vi "Manual Mode(orig).vi"(5 "slider shoot":dbl, 6 "4 and 5":cluster{"Button 4":bool, "Button 5":bool}, 7 "Shooter":T1, 8 "engage shoot":bool, 9 "Potent":dbl, 11 "Button 1":bool) -> ()   [LabVIEW 2012]
uses:
  <vilib>/Platform/TimedLoop/XDataNode/timing_clust.ctl
  <vilib>/Platform/TimedLoop/XDataNode/nitl_modes.ctl
  <vilib>/Platform/TimedLoop/XDataNode/wakeup.ctl
  <vilib>/Rock Robotics/WPI/Solenoid/WPI_SolenoidValue.ctl
  <vilib>/Rock Robotics/WPI/Joystick/WPI_JoystickGetSetRefNum.vi
  <vilib>/Rock Robotics/WPI/RobotDrive/WPI_RobotDriveArcadeDrive_Standard(NoSaturation).vi
  <vilib>/Rock Robotics/WPI/RobotDrive/WPI_RobotDriveGetSetRefNum.vi
  <vilib>/Rock Robotics/WPI/Solenoid/WPI_SolenoidSetEnum.vi
  <vilib>/platform/TimedLoop/XDataNode/XDataNode.xnode
  <vilib>/Platform/TimedLoop/XDataNode/XDNodeRunTimeDep.lvlib
panel:
  out "seconds calc":dbl
  out "seconds":dbl
  in  "speed":dbl
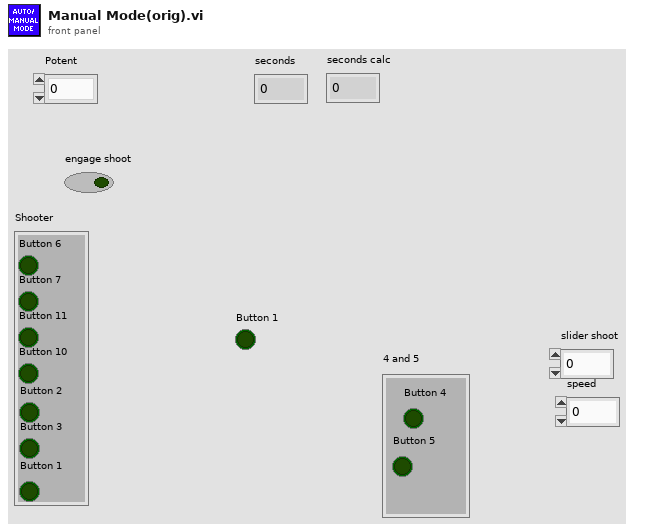
[diagram p1: front panel]
types:
  T1 = cluster{"Button 6":bool, "Button 7":bool, "Button 11":bool, "Button 10":bool, "Button 2":bool, "Button 3":bool, "Button 1":bool}
  T2 = typedef "WPI_JoystickDevRef.ctl" = cluster{"Device":T3}
  T3 = typedef "WPI_JoystickDeviceEnum.ctl" = enum16{"USB 1", "USB 2", "USB 3", "USB 4", "Kinect 1", "Kinect 2"}
  T4 = typedef "WPI_MotorControlDeviceRef.ctl" = cluster{"DeviceStatus":errorcluster, "Type":enum16{"PWM", "CAN"}, "PWM":cluster{"Digital Module":T5, "PWM Channel":T6, "DeadBand":T7}, "CAN":cluster{"Device Number":u8, "Control Mode":T8, "Semaphore":T9, "Max Vout":dbl}, "Invert":bool, "TransformRef":T10, "InvTransformRef":T10}
  T5 = typedef "FPGA_TypedefDigitalModule.ctl" = enum16{"Digital Module 1", "Digital Module 2"}
  T6 = typedef "FPGA_DIOPWMChannel.ctl" = enum8{"PWM 1", "PWM 2", "PWM 3", "PWM 4", "PWM 5", "PWM 6", "PWM 7", "PWM 8", "PWM 9", "PWM 10", "Invalid"}
  T7 = typedef "WPI_PWMDeadband.ctl" = cluster{"Name":string, "maxPositivePwm":i32, "minPositivePwm":i32, "centerPwm":i32, "maxNegativePwm":i32, "minNegativePwm":i32, "angularRange":u16}
  T8 = typedef "WPI_CANJaguar_ControlMode.ctl" = enum8{"Percent VBus", "Current", "Speed", "Position", "Voltage"}
  T9 = typedef "Semaphore RefNum" = refnum<k1>
  T10 = typedef "WPI_PWMTransform_ConPane.ctl" = refnum<vi>
  T11 = typedef "WPI_SolenoidDevRef.ctl" = cluster{"DevStatus":errorcluster, "Solenoid Module":T12, "Forward Solenoid Channel":T13, "Reverse Solenoid Channel":T13}
  T12 = typedef "FPGA_TypedefSolenoidModule.ctl" = enum16{"Solenoid Module 1", "Solenoid Module 2"}
  T13 = typedef "WPI_SolenoidChannel.ctl" = enum8{"Solenoid 1", "Solenoid 2", "Solenoid 3", "Solenoid 4", "Solenoid 5", "Solenoid 6", "Solenoid 7", "Solenoid 8", "Invalid"}
  T14 = typedef "WPI_JoystickButtonState.ctl" = cluster{"Button 1":bool, "Button 2":bool, "Button 3":bool, "Button 4":bool, "Button 5":bool, "Button 6":bool, "Button 7":bool, "Button 8":bool, "Button 9":bool, "Button 10":bool, "Button 11":bool, "Button 12":bool}
  T15 = typedef "XDNodeRunTimeDep.lvlib/timing_clust.ctl" = cluster{"Expected End [f-1]":u64, "Actual End [f-1]":u64, "Finished Late? [f-1]":bool, "Expected End [i-1]":u64, "Actual End [i-1]":u64, "Finished Late? [i-1]":bool, "Expected Start [i]":u64, "Actual Start [i]":u64, "Expected Start [f]":u64, "Actual Start [f]":u64, "Source Name":string, "Structure Name":string, "Period":i64, "Deadline":i64, "Offset":i64, "Start":i64, "Priority":i32, "Timeout":i32, "Mode":T16, "Wakeup Reason":T17, "Error":errorcluster, "Source Type":string, "Secondary Source Type":string, "Global End Time":u64, "Global Start Time":u64, "Frame Duration":u64, "Iteration Duration":u64, "Assigned CPU":i32, "I/O Scan Engine Mode":u32}
  T16 = typedef "XDNodeRunTimeDep.lvlib/nitl_modes.ctl" = enum32{"No Change", "Process missed periods, maintain original phase", "Discard missed periods, maintain original phase", "Process missed periods, ignore original phase", "Discard missed periods, ignore original phase"}
  T17 = typedef "XDNodeRunTimeDep.lvlib/wakeup.ctl" = enum32{"Normal", "Aborted", "Asynchronous wakeup", "Timing source error", "Timed loop error", "Timeout"}
  T18 = typedef "WPI_SolenoidValue.ctl" = enum16{"Off", "On", "Forward", "Reverse"}
  T19 = typedef "WPI_AnalogChannelDevRef.ctl" = cluster{"DevStatus":errorcluster, "Analog Module":T20, "Analog Channel":T21}
  T20 = typedef "FPGA_TypedefAnalogModule.ctl" = enum16{"Analog Module 1", "Analog Module 2"}
  T21 = typedef "FPGA_AIChannel.ctl" = enum8{"AI 1", "AI 2", "AI 3", "AI 4", "AI 5", "AI 6", "AI 7", "AI 8", "Invalid"}
  T22 = typedef "WPI_RobotDriveDevRef.ctl" = cluster{"DevStatus":errorcluster, "Motors[]":T4[], "Square Inputs":bool, "Max Output":dbl, "Isochronous":bool}
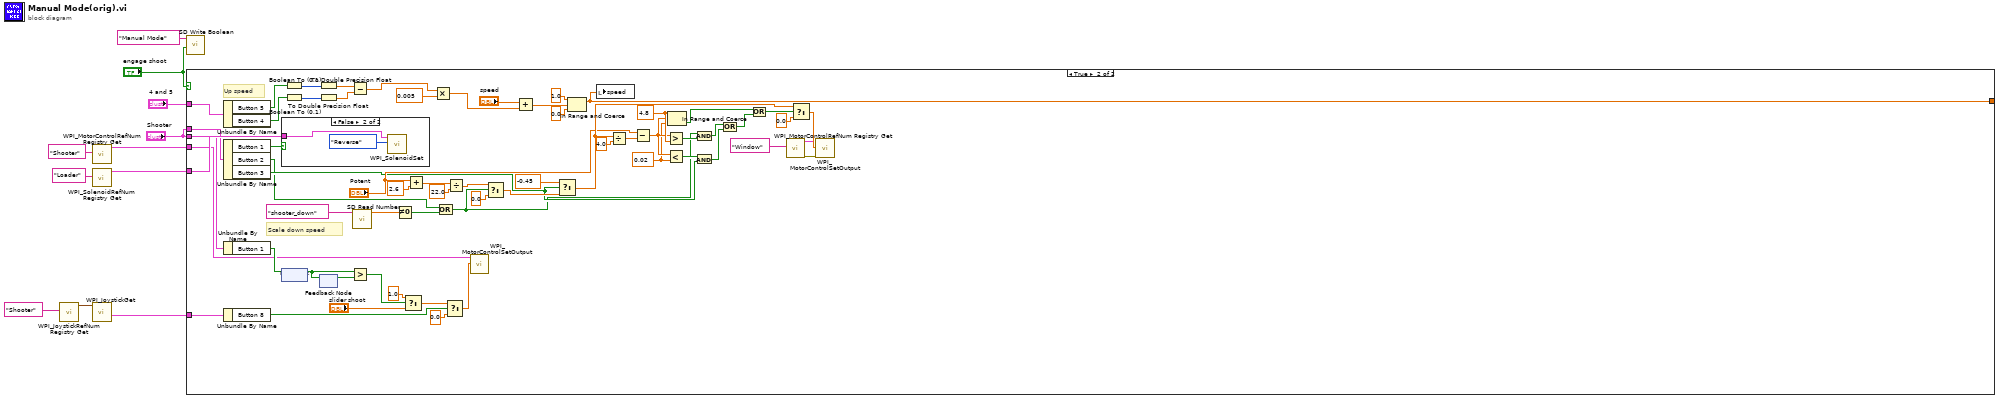
[diagram p0: block diagram]
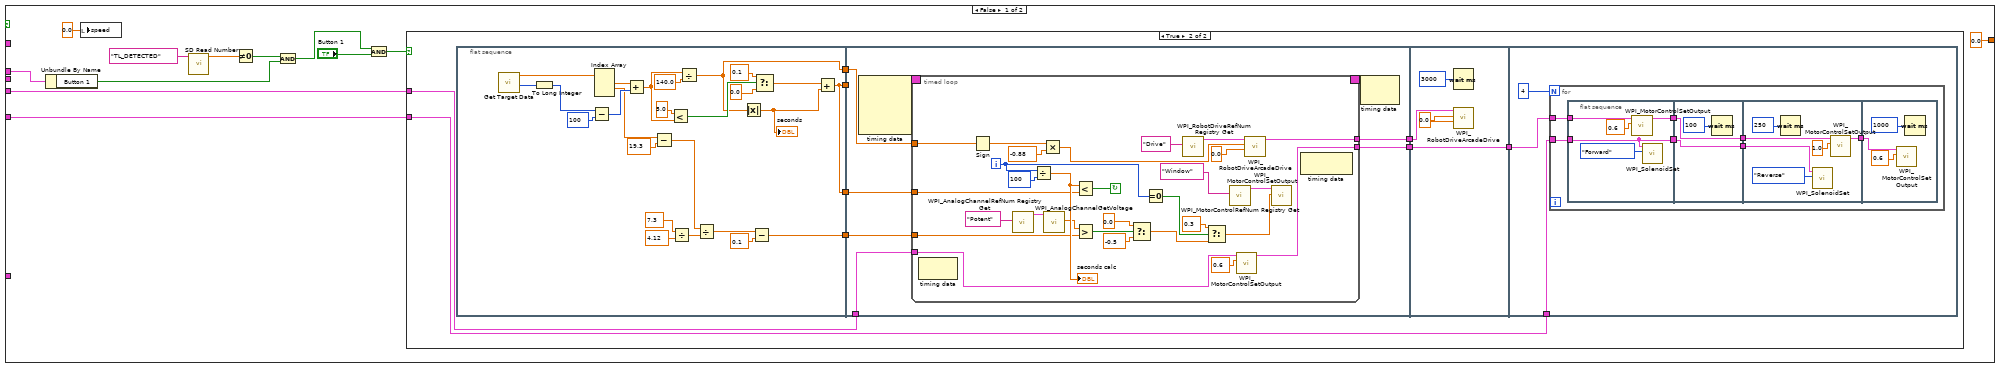
[diagram p2: hidden frame]
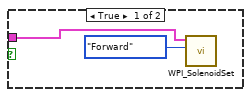
[diagram p4: hidden frame]
diagram:
  n1 = call <vilib>:"WPI_JoystickRefNum Registry Get.vi"("refnum name"="Shooter") -> ("JoystickDevRef"=w5:T2)  [unwired: 9 in, 1 out]
  n2 = call <vilib>:"WPI_MotorControlRefNum Registry Get.vi"("refnum name"="Shooter") -> ("MotorControlDevRef"=w3:T4)  [unwired: 9 in, 1 out]
  n3 = call <vilib>:"WPI_SolenoidRefNum Registry Get.vi"("refnum name"="Loader") -> ("SolenoidDevRef"=w10:T11)  [unwired: 9 in, 1 out]
  n4 = call <vilib>:"WPI_JoystickGet.vi"("JoystickDevRef"=w5) -> ("Buttons"=w2:T14)  [unwired: 4 in, 2 out]
  n5 = call <vilib>:"SD Write Boolean.vi"("Boolean"="engage shoot", "Name"="Manual Mode") -> ()  [unwired: 8 in, 2 out]
  n6 = case shown="True" "engage shoot" {
    tunnel: "Shooter" -> [w23 w158]
    tunnel: w10 -> [w18 w164]
    tunnel: "4 and 5" -> [_ w153]
    tunnel: [0.0 ("upper limit") w148] -> _
    tunnel: w3 -> [w12 w137]
    tunnel: w2 -> [_ w136]
    tunnel: "Shooter" -> [_ w135]
    frame False {
      n7 = Unbundle By Name(w23) -> ("Button 1"=w17:bool)
      n8 = local write "speed"(0.0 ("speed")) -> ()
      n9 = call <vilib>:"SD Read Number.vi"("Name"="TL_DETECTED") -> ("Numeric"=w13:dbl)  [unwired: 8 in, 2 out]
      n10 = Not Equal To 0?(x=w13) -> (x != 0?=w14:bool)
      n11 = And(x=w14, y=w17) -> (x .and. y?=w16:bool)
      n12 = And(x=w16, y="Button 1") -> (x .and. y?=w22:bool)
      n13 = case shown="True" w22 {
        tunnel: w18 -> [_ w32]
        tunnel: w12 -> [_ w29]
        frame False {
        }
        frame True {
          n14 = flat-sequence {
            tunnel: [w50] -> w28
            tunnel: [w50] -> w27
            tunnel: [w35] -> w25
            tunnel: [w33] -> w24
            tunnel: [w65] -> w31
            tunnel: w29 -> [w62]
            tunnel: w28 -> [_]
            tunnel: w27 -> [w61]
            tunnel: [w60] -> w26
            tunnel: w25 -> [w59]
            tunnel: w24 -> [w58]
            tunnel: w31 -> [w102]
            tunnel: [w102] -> w30
            tunnel: w26 -> [w99]
            tunnel: w32 -> [w104]
            tunnel: w30 -> [w103]
            frame #0 {
              n15 = call "Get Target Data.vi"() -> ("x angle"=w52:u16, "values"=w56:dbl[])  [unwired: 9 in, 1 out]
              n16 = To Long Integer(number=w52) -> (32bit integer=w53:i32)
              n17 = Subtract(x=w53, y=100) -> (x-y=w55:i32)
              n18 = Index Array(array=w56) -> (element #1=w54:dbl, element #2=w44:dbl)  [unwired: 3 in, 1 out]
              n19 = Add(x=w54, y=w55) -> (x+y=w45:dbl)
              n20 = Subtract(x=w44, y=19.3) -> (x-y=w41:dbl)
              n21 = Less?(x=5.0, y=w45) -> (x < y?=w46:bool)
              n22 = Divide(x=7.3, y=4.12) -> (x/y=w40:dbl)
              n23 = Divide(x=w45, y=140.0) -> (x/y=w33:dbl)
              n24 = Divide(x=w41, y=w40) -> (x/y=w37:dbl)
              n25 = Absolute Value(x=w33) -> (abs(x)=w34:dbl)
              "seconds" <- w34
              n26 = Subtract(x=w37, y=0.1) -> (x-y=w35:dbl)
              n27 = Select(t=0.1 ("x"), s=w46, f=0.0) -> (s? t:f=w48:dbl)
              n28 = Add(x=w48, y=w34) -> (x+y=w50:dbl)
            }
            frame #1 {
              n29 = node-c288() -> (w64:T15)  [unwired: 4 in]
              n30 = timed-loop {
                timing: w64 -> [_]
                timing-out: [_] -> w63
                tunnel: [w89] -> w65
                tunnel: w62 -> [w91]
                tunnel: w58 -> [w88]
                tunnel: w61 -> [w90]
                tunnel: [w81] -> w60
                tunnel: w59 -> [w71]
                i -> [w80]
                stop <- w94 continue-if-true
                n31 = node-c288() -> ()  [unwired: 1 in, 1 out]
                n32 = Sign(1:w88) -> (0:w87:dbl)
                n33 = call <vilib>:"WPI_AnalogChannelRefNum Registry Get.vi"("refnum name"="Potent") -> ("AIDeviceRef"=w72:T19)  [unwired: 9 in, 1 out]
                n34 = Divide(x=w80, y=100) -> (x/y=w92:dbl)
                "seconds calc" <- w92
                n35 = Multiply(x=w87, y=-0.88) -> (x*y=w84:dbl)
                n36 = call <vilib>:"WPI_AnalogChannelGetVoltage.vi"("AIDeviceRef"=w72) -> ("Voltage"=w70:dbl)  [unwired: 8 in, 2 out]
                n37 = Less?(x=w92, y=w90) -> (x < y?=w94:bool)
                n38 = Greater?(x=w70, y=w71) -> (0:w69:bool)
                n39 = Select(t=0.0, s=w69, f=-0.5) -> (s? t:f=w66:dbl)
                n40 = Equal To 0?(x=w80) -> (x = 0?=w77:bool)
                n41 = call <vilib>:"WPI_RobotDriveRefNum Registry Get.vi"("refnum name"="Drive") -> ("RobotDriveDevRef"=w85:T22)  [unwired: 9 in, 1 out]
                n42 = Select(t=0.3, s=w77, f=w66) -> (s? t:f=w76:dbl)
                n43 = call <vilib>:"WPI_MotorControlRefNum Registry Get.vi"("refnum name"="Window") -> ("MotorControlDevRef"=w78:T4)  [unwired: 9 in, 1 out]
                n44 = call <vilib>:"WPI_MotorControlSetOutput.vi"("Output"=0.6, "MotorControlDevRef"=w91) -> ("MotorControlDevRef"=w89:T4)  [unwired: 7 in, 2 out]
                n45 = call-poly <vilib>:"WPI_RobotDriveArcadeDrive.vi"("Y axis value"=0.0, "X axis value"=w84, "RobotDriveDevRef"=w85) -> ("RobotDriveDevRef"=w81:T22)  [unwired: 6 in, 2 out]
                n46 = call <vilib>:"WPI_MotorControlSetOutput.vi"("Output"=w76, "MotorControlDevRef"=w78) -> ()  [unwired: 7 in, 3 out]
                n47 = node-c288() -> ()  [unwired: 1 in, 1 out]
              }
              n48 = node-c288(w63) -> ()  [unwired: 1 out]
            }
            frame #2 {
              w100 = 0.0 ("X axis value")
              n49 = Wait (ms)(milliseconds to wait=u32 3000) -> ()  [unwired: 1 out]
              n50 = call-poly <vilib>:"WPI_RobotDriveArcadeDrive.vi"("Y axis value"=w100, "X axis value"=w100, "RobotDriveDevRef"=w99) -> ()  [unwired: 6 in, 3 out]
            }
            frame #3 {
              n51 = for {
                N: 4 -> [_]
                tunnel: w104 -> [w112]
                tunnel: w103 -> [w109]
                n52 = flat-sequence {
                  tunnel: w112 -> [w116]
                  tunnel: [w116] -> w111
                  tunnel: w109 -> [w114]
                  tunnel: [w113] -> w107
                  tunnel: w111 -> [w120]
                  tunnel: [w120] -> w110
                  tunnel: [w118] -> w108
                  tunnel: w107 -> [w118]
                  tunnel: w110 -> [w125]
                  tunnel: w108 -> [w123]
                  tunnel: [w122] -> w106
                  tunnel: w106 -> [w128]
                  frame #0 {
                    n53 = call <vilib>:"WPI_MotorControlSetOutput.vi"("Output"=0.6, "MotorControlDevRef"=w114) -> ("MotorControlDevRef"=w113:T4)  [unwired: 7 in, 2 out]
                    n54 = call-poly <vilib>:"WPI_SolenoidSet.vi"("Value"=WPI_SolenoidValue."Forward", "SolenoidDevRef"=w116) -> ()  [unwired: 8 in, 2 out]
                  }
                  frame #1 {
                    n55 = Wait (ms)(milliseconds to wait=u32 100) -> ()  [unwired: 1 out]
                  }
                  frame #2 {
                    n56 = Wait (ms)(milliseconds to wait=u32 250) -> ()  [unwired: 1 out]
                    n57 = call-poly <vilib>:"WPI_SolenoidSet.vi"("Value"=WPI_SolenoidValue."Reverse", "SolenoidDevRef"=w125) -> ()  [unwired: 8 in, 2 out]
                    n58 = call <vilib>:"WPI_MotorControlSetOutput.vi"("Output"=1.0, "MotorControlDevRef"=w123) -> ("MotorControlDevRef"=w122:T4)  [unwired: 7 in, 2 out]
                  }
                  frame #3 {
                    n59 = call <vilib>:"WPI_MotorControlSetOutput.vi"("Output"=0.6, "MotorControlDevRef"=w128) -> ()  [unwired: 7 in, 3 out]
                    n60 = Wait (ms)(milliseconds to wait=u32 1000) -> ()  [unwired: 1 out]
                  }
                }
              }
            }
          }
        }
      }
    }
    frame True {
      w172 = 0.02 ("lower limit")
      w177 = 4.8 ("upper limit")
      # "Scale down speed"
      # "Up speed"
      n61 = Unbundle By Name(w153) -> ("Button 5"=w152:bool, "Button 4"=w151:bool)
      n62 = Unbundle By Name(w158) -> ("Button 1"=w165:bool, "Button 2"=w132:bool, "Button 3"=w166:bool)
      n63 = Unbundle By Name(w135) -> ("Button 1"=w144:bool)
      n64 = Unbundle By Name(w136) -> ("Button 8"=w140:bool)
      n65 = case shown="False" w165 {
        tunnel: w164 -> [w193 w195]
        frame True {
          n66 = call-poly <vilib>:"WPI_SolenoidSet.vi"("Value"=WPI_SolenoidValue."Forward", "SolenoidDevRef"=w193) -> ()  [unwired: 8 in, 2 out]
        }
        frame False {
          n67 = call-poly <vilib>:"WPI_SolenoidSet.vi"("Value"=WPI_SolenoidValue."Reverse", "SolenoidDevRef"=w195) -> ()  [unwired: 8 in, 2 out]
        }
      }
      n68 = feedback #1() -> (w146:bool)  [unwired: 1 in]
      n69 = feedback-in #1(w144) -> ()
      n70 = Boolean To (0,1)(Boolean=w152) -> (0, 1=w157:i16)
      n71 = Boolean To (0,1)(Boolean=w151) -> (0, 1=w155:i16)
      n72 = To Double Precision Float(number=w157) -> (double precision float=w156:dbl)
      n73 = To Double Precision Float(number=w155) -> (double precision float=w154:dbl)
      n74 = feedback #2() -> (w147:bool)  [unwired: 1 in]
      n75 = feedback-in #2(w146) -> ()
      n76 = Subtract(x=w156, y=w154) -> (x-y=w163:dbl)
      n77 = Greater?(x=w146, y=w147) -> (0:w145:bool)
      n78 = call <vilib>:"SD Read Number.vi"("Name"="shooter_down") -> ("Numeric"=w134:dbl)  [unwired: 8 in, 2 out]
      n79 = Not Equal To 0?(x=w134) -> (x != 0?=w131:bool)
      n80 = Select(t=1.0, s=w145, f="slider shoot") -> (s? t:f=w141:dbl)
      n81 = Add(x="Potent", y=2.6) -> (x+y=w181:dbl)
      n82 = Multiply(x=w163, y=0.005) -> (x*y=w161:dbl)
      n83 = Or(x=w132, y=w131) -> (x .or. y?=w130:bool)
      n84 = Select(t=w141, s=w140, f=0.0) -> (s? t:f=w138:dbl)
      n85 = Divide(x=w181, y=22.0) -> (x/y=w178:dbl)
      n86 = call <vilib>:"WPI_MotorControlSetOutput.vi"("Output"=w138, "MotorControlDevRef"=w137) -> ()  [unwired: 7 in, 3 out]
      n87 = Select(t=w178, s=w130, f=0.0) -> (s? t:f=w176:dbl)
      n88 = Add(x="speed", y=w161) -> (x+y=w159:dbl)
      n89 = Select(t=-0.45, s=w166, f=w176) -> (s? t:f=w185:dbl)
      n90 = In Range and Coerce(upper limit=1.0, x=w159, lower limit=0.0) -> (coerced(x)=w148:dbl)  [unwired: 1 out]
      n91 = local write "speed"(w148) -> ()
      n92 = Divide(x=w185, y=4.0) -> (x/y=w184:dbl)
      n93 = Subtract(x="Potent", y=w184) -> (x-y=w173:dbl)
      n94 = Greater?(x=w173, y=w177) -> (0:w175:bool)
      n95 = Less?(x=w173, y=w172) -> (x < y?=w171:bool)
      n96 = In Range and Coerce(upper limit=w177, x=w173, lower limit=w172) -> (In Range?=w167:bool)  [unwired: 1 out]
      n97 = And(x=w130, y=w175) -> (x .and. y?=w174:bool)
      n98 = And(x=w171, y=w166) -> (x .and. y?=w168:bool)
      n99 = Or(x=w174, y=w168) -> (x .or. y?=w170:bool)
      n100 = Or(x=w167, y=w170) -> (x .or. y?=w169:bool)
      n101 = call <vilib>:"WPI_MotorControlRefNum Registry Get.vi"("refnum name"="Window") -> ("error out"=w186:errorcluster, "MotorControlDevRef"=w187:T4)  [unwired: 9 in]
      n102 = Select(t=w185, s=w169, f=0.0) -> (s? t:f=w188:dbl)
      n103 = call <vilib>:"WPI_MotorControlSetOutput.vi"("error in (no error)"=w186, "Output"=w188, "MotorControlDevRef"=w187) -> ()  [unwired: 6 in, 3 out]
    }
  }
